vi "Apply Channel.vi"(8 "error in":errorcluster, 11 "2727 in":refnum<class "2727.lvclass">) -> (0 "error out":errorcluster, 3 "2727 out":refnum<class "2727.lvclass">)   [LabVIEW 2019, in "2727.lvlib" / "2727.lvclass"]
uses:
  Library/2727.lvclass
  C:/Users/Public/Documents/Development/builds/Instruments/PRM.lvlibp/Library/PRM.lvclass
  Library/2727.lvclass/2727.ctl
  builds/Instruments/PRM.lvlibp/Accessors/Read Active Channel.vi
  builds/Instruments/PRM.lvlibp/Accessors/Read Setting.vi
  builds/Instruments/PRM.lvlibp/Accessors/Read Units.vi
  builds/Instruments/PRM.lvlibp/Accessors/Read RTD_Parameter.vi
  <instrlib>/ni272xReferenceVIs/ni272xReferenceVIs.llb/ni272x Write Resistance 1Chan 1Samp.vi
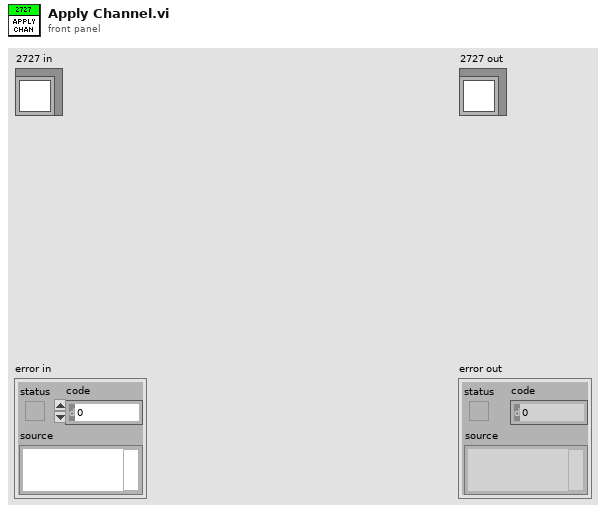
[diagram p1: front panel]
types:
  T1 = typedef "PRM.lvlibp/PRM.lvclass/Units.ctl" = enum16{"Celsius", "Fahrenheit", "Kelvin", "Ohms"}
  T2 = typedef "PRM.lvlibp/PRM.lvclass/RTD Parameters.ctl" = cluster{"A":dbl, "B":dbl, "C":dbl, "R0":dbl}
  T3 = typedef "ni272x Reference.ctl" = refnum<k20>
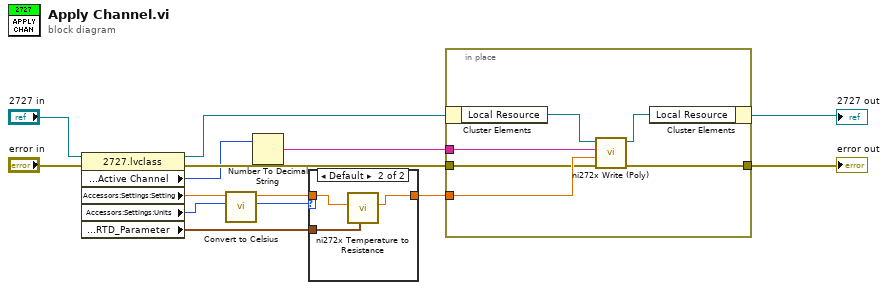
[diagram p0: block diagram]
diagram:
  n1 = property class="2727.lvclass"(reference="2727 in", error in="error in") -> (reference out=w10:refnum<class "2727.lvclass">, error out=w4:errorcluster, "Accessors:Settings:Active Channel"=w2:u32, "Accessors:Settings:Setting"=w12:dbl, "Accessors:Settings:Units"=w11:T1, "Accessors:Config:RTD_Parameter"=w6:T2)
  n2 = call "Convert to Celsius.vi"("Units in"=w11, "Value in"=w12) -> ("Units out"=w8:T1, "Value out"=w7:dbl)  [unwired: 8 in]
  n3 = Number To Decimal String(number=w2) -> (decimal integer string=w1:string)  [unwired: 1 in]
  n4 = case shown="Default" w8 {
    tunnel: w7 -> [w15 w18]
    tunnel: w6 -> [_ w16]
    tunnel: [w15 w17] -> w5
    frame "Ohms" {
    }
    frame Default {
      n5 = call <instrlib>:"ni272x Temperature to Resistance.vi"("Callendar-Van Dusen RTD parameters"=w16, "temperature (degrees Celsius)"=w18) -> ("resistance (ohms)"=w17:dbl)  [unwired: 9 in]
    }
  }
  n6 = in-place {
    in-place-border: w5 -> [w22]
    in-place-border: w4 -> [w21]
    in-place-border: [w20] -> w3
    in-place-border: w1 -> [w19]
    n7 = in-place-cluster #1(w10) -> ("Local Resource"=w24:T3)
    n8 = call-poly <instrlib>:"ni272x Write (Poly).vi"("error in (no error)"=w21, "requested resistance (ohms)"=w22, "resistor channel"=w19, "instrument handle"=w24) -> ("error out"=w20:errorcluster, "instrument handle out"=w23:T3)  [unwired: 1 in, 5 out]
    n9 = in-place-cluster #1("Local Resource"=w23) -> (→"2727 out":refnum<class "2727.lvclass">)
  }
  "error out" <- w3
